vi "Read Duration MM.vi"(8 "error in (no error)":errorcluster, 11 "Acquis params in":refnum<class "CV-Acquisition.lvclass">) -> (0 "error out":errorcluster, 2 "Duration MM":sgl min=0 max=59 step=1 format="%02.0f", 3 "Acquis params out":refnum<class "CV-Acquisition.lvclass">)   [LabVIEW 2013, in "CameraVision.lvlib" / "CV-Acquisition.lvclass"]
uses:
  CV-Acquisition.lvclass
  CV-Acquisition.lvclass/CV-Acquisition.ctl
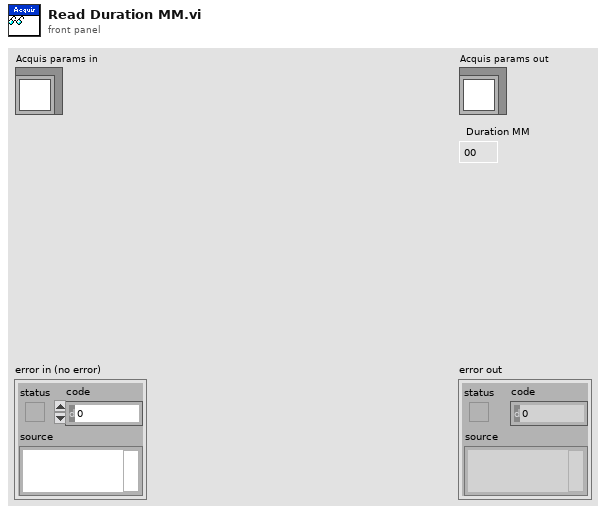
[diagram p1: front panel]
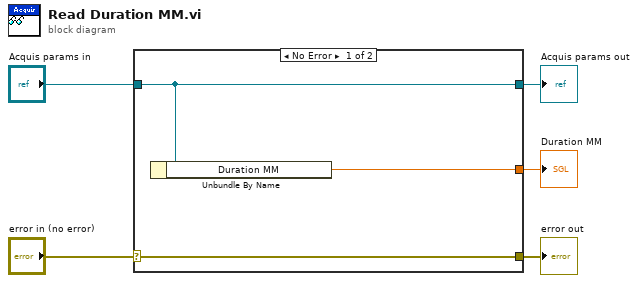
[diagram p0: block diagram]
diagram:
  n1 = case shown="No Error" "error in (no error)" {
    selector: "error in (no error)" -> [w8 w9]
    tunnel: [w8 w9] -> w4
    tunnel: [w7 w10] -> w2
    tunnel: "Acquis params in" -> [w7 w10]
    tunnel: [w6 _] -> w1
    frame No Error {
      n2 = Unbundle By Name(w7) -> ("Duration MM"=w6:sgl)
    }
    frame Error {
    }
  }
  "error out" <- w4
  "Acquis params out" <- w2
  "Duration MM" <- w1
